vi "WriteDataBDD.vi"(8 "errin":errorcluster, 9 "table":string, 10 "data":string[](array[string]), 11 "id":string[](array[string])) -> (0 "error out":errorcluster, 3 "requette":string)   [LabVIEW 2020]
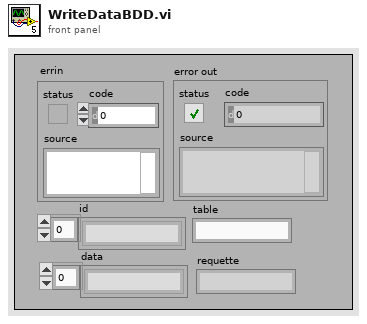
[diagram p1: front panel]
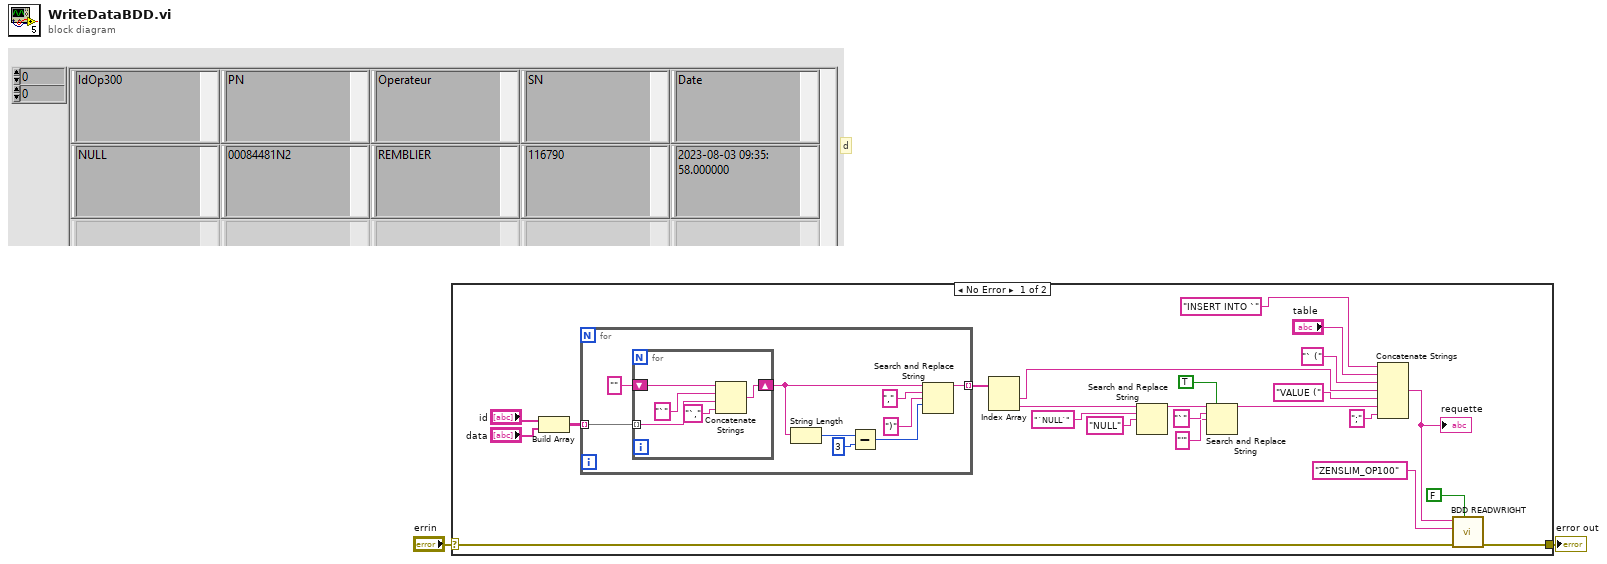
[diagram p0: block diagram]
diagram:
  # "d"
  n1 = case shown="No Error" "errin" {
    selector: "errin" -> [w24 w40]
    tunnel: [w25 w40] -> w2
    frame No Error {
      n2 = Build Array("id", "data") -> (w23:string[][])
      n3 = for {
        tunnel: [w26] -> w5 mode=indexing
        tunnel: w23 -> [w34] mode=indexing
        n4 = for {
          shift-right: [w37] -> w27
          shift-left: "" -> [w36]
          tunnel: w34 -> [w35] mode=indexing
          n5 = Concatenate Strings(w36, "`" ("string"), w35, "`," ("string")) -> (w37:string)
        }
        n6 = String Length(string=w27) -> (length=w32:i32)
        n7 = Subtract(x=w32, y=3) -> (x-y=w30:i32)
        n8 = Search and Replace String(input string=w27, search string=",", replace string=")" ("replace string (\"\")"), offset=w30) -> (result string=w26:string)  [unwired: 4 in, 3 out]
      }
      n9 = Index Array(array=w5) -> (element #1=w18:string, element #2=w20:string)  [unwired: 2 in]
      n10 = Search and Replace String(input string=w20, search string="`NULL`", replace string="NULL" ("replace string (\"\")")) -> (result string=w21:string)  [unwired: 5 in, 3 out]
      n11 = Search and Replace String(replace all?=TRUE ("replace all? (F)"), input string=w21, search string="`", replace string="'" ("replace string (\"\")")) -> (result string=w22:string)  [unwired: 4 in, 3 out]
      n12 = Concatenate Strings("INSERT INTO `" ("string"), "table", "` (" ("string"), w18, "VALUE (" ("string"), w22, ";" ("string")) -> (w19:string)
      "requette" <- w19
      n13 = call <userlib>:"BDD READWRIGHT.vi"("Read?"=FALSE, "errin"=w24, "DSN name"="ZENSLIM_OP100", "Instruction"=w19) -> ("error out"=w25:errorcluster)  [unwired: 6 in, 1 out]
    }
    frame Error {
    }
  }
  "error out" <- w2
